vi "Verify LEUI Binary Blinking.vi"(0 "GEA2 Reference In":refnum<k24>, 1 "Standalone":bool, 2 "Initial Timeout (s)":dbl, 5 "Numeric":u8, 7 "Retry Count":i32, 9 "Max Blink Rate (sec)":dbl, 11 "Error In":errorcluster, 12 "Ignore Brightness":bool) -> (4 "GEA2 Reference Out":refnum<k24>, 6 "Pass/Fail?":bool, 10 "Report Text":string, 14 "Blink Times (s)":dbl[](array[numeric]), 15 "Error Out":errorcluster)   [LabVIEW 2016, in "Centauro.lvlib"]
uses:
  Projects/Centauro.lvlib
  Q:/Common/DLLs/GEA3/GeaCommunication.dll
  Common/DLLs/GEA3/GeaCommunication.dll
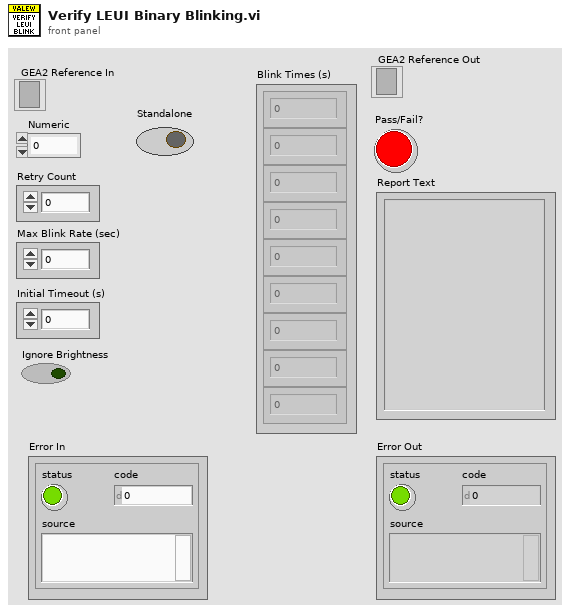
[diagram p1: front panel]
types:
  T1 = cluster{"Deep Rinse":bool, "Wash":bool, "Rinse":bool, "Spin":bool, "Lid Lock":bool}
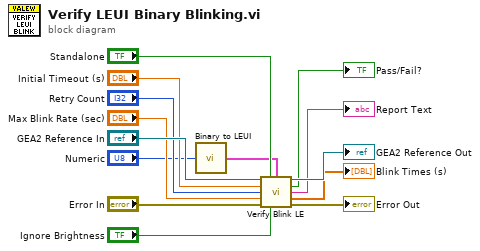
[diagram p0: block diagram]
diagram:
  n1 = call "Binary to LEUI.vi"("Numeric"="Numeric") -> ("Blinking Out"=w1:T1)  [unwired: 14 in]
  n2 = call "Verify Blink LE.vi"("GEA2 Reference In"="GEA2 Reference In", "Standalone"="Standalone", "Blinking LED"=w1, "Initial Timeout (s)"="Initial Timeout (s)", "Retry Count"="Retry Count", "Max Blink Rate (sec)"="Max Blink Rate (sec)", "Error In"="Error In", "Ignore Brightness"="Ignore Brightness") -> ("GEA2 Reference Out"=→"GEA2 Reference Out":refnum<k24>, "Pass/Fail?"=→"Pass/Fail?":bool, "Report Text"=→"Report Text":string, "Blink Times (s)"=→"Blink Times (s)":dbl[], "Error Out"=→"Error Out":errorcluster)  [unwired: 2 in, 1 out]
